vi "get value.vi"(8 "error in (no error)":errorcluster, 11 "JSON string":string) -> (0 "error out":errorcluster, 3 "value":string)   [LabVIEW 2020, in "ui-testing.lvlib"]
uses:
  ui-testing.lvlib
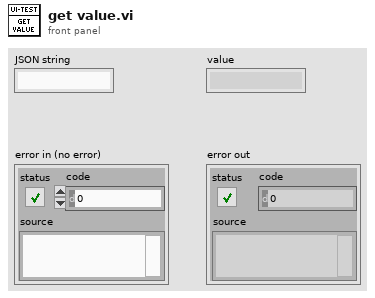
[diagram p1: front panel]
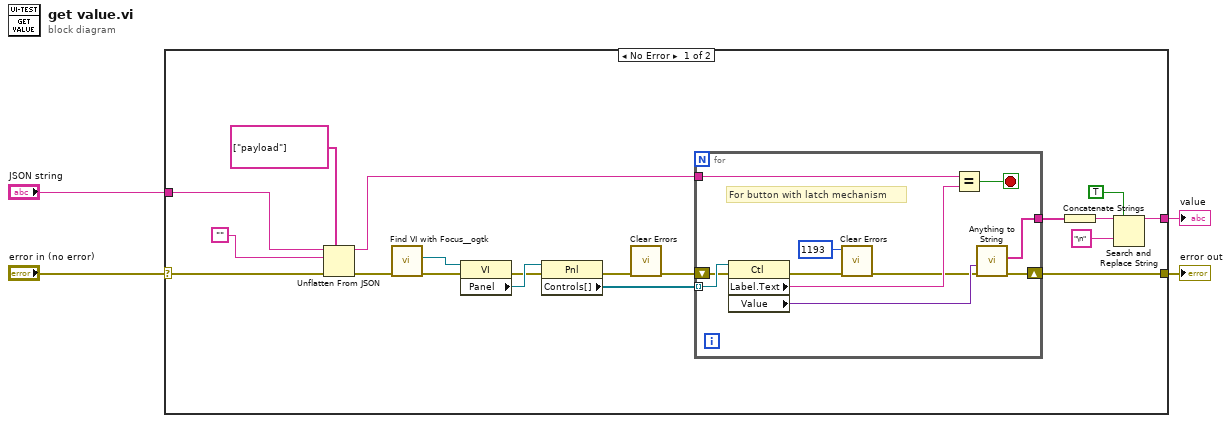
[diagram p0: block diagram]
diagram:
  n1 = case shown="No Error" "error in (no error)" {
    selector: "error in (no error)" -> [w9 w35]
    tunnel: "JSON string" -> [w13 _]
    tunnel: [w10 w35] -> w3
    tunnel: [w7 _] -> w2
    frame No Error {
      n2 = Unflatten From JSON(path=string[] ["payload"], JSON string=w13, type and defaults="", error in (no error)=w9) -> (value=w16:string, error out=w17:errorcluster)  [unwired: 3 in]
      n3 = call <userlib>:"Find VI with Focus__ogtk.vi"("error in"=w17) -> ("error out"=w22:errorcluster, "VI with Focus"=w21:refnum<vi>)  [unwired: 6 in, 3 out]
      n4 = property class="VI"(reference=w21, error in=w22) -> (error out=w18:errorcluster, "Panel"=w20:refnum<vi>)  [unwired: 1 out]
      n5 = property class="Pnl"(reference=w20, error in=w18) -> (error out=w12:errorcluster, "Controls[]"=w19:refnum<vi>[])  [unwired: 1 out]
      n6 = call <vilib>:"Clear Errors.vi"("error in (no error)"=w12) -> ("error out"=w11:errorcluster)  [unwired: 5 in, 1 out]
      n7 = for {
        tunnel: w19 -> [w34] mode=indexing
        tunnel: w16 -> [w32]
        tunnel: [w29] -> w15
        shift-right: [w24] -> w10
        shift-left: w11 -> [w26]
        stop <- w31 stop-if-true
        # "For button with latch mechanism"
        n8 = property class="Ctl"(reference=w34, error in=w26) -> (error out=w28:errorcluster, "Label.Text"=w33:string, "Value"=w30:variant)  [unwired: 1 out]
        n9 = call <vilib>:"Clear Errors.vi"("error in (no error)"=w28, "specific error code to clear (0: all)"=1193) -> ("error out"=w25:errorcluster)  [unwired: 4 in, 1 out]
        n10 = Equal?(x=w32, y=w33) -> (x = y?=w31:bool)
        n11 = call <userlib>:"Anything to String.vi"("Error In"=w25, "Anything"=w30) -> ("Error Out"=w24:errorcluster, "Strings[]"=w29:string[])  [unwired: 7 in, 1 out]
      }
      n12 = Concatenate Strings(w15) -> (w8:string)
      n13 = Search and Replace String(replace all?=TRUE ("replace all? (F)"), input string=w8, search string="\n") -> (result string=w7:string)  [unwired: 5 in, 3 out]
    }
    frame Error {
    }
  }
  "error out" <- w3
  "value" <- w2
